vi "Create All Message Queues.vi"(8 "error in (no error)":errorcluster) -> (0 "error out":errorcluster, 3 "Message Queues out":T1)   [LabVIEW 2015, in "Message Queue.lvlib"]
doc: "This VI creates and initializes all the message queues for your application. If your application requires more than one message queue, right-click the \"Message Queues\" constant above and select Open Type Def. Add the new Message Queue(s) to the type definition, then initialize them in this VI."
uses:
  Message Queue.lvlib
  All Message Queues.ctl
  Message Cluster.ctl
  Enqueue Message (Single).vi
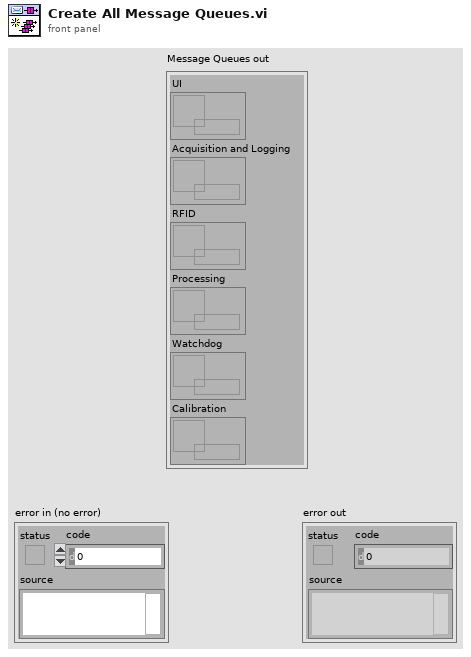
[diagram p1: front panel]
types:
  T1 = typedef "Message Queue.lvlib/All Message Queues.ctl" = cluster{"UI":refnum<queue>, "Acquisition and Logging":refnum<queue>, "RFID":refnum<queue>, "Processing":refnum<queue>, "Watchdog":refnum<queue>, "Calibration":refnum<queue>}
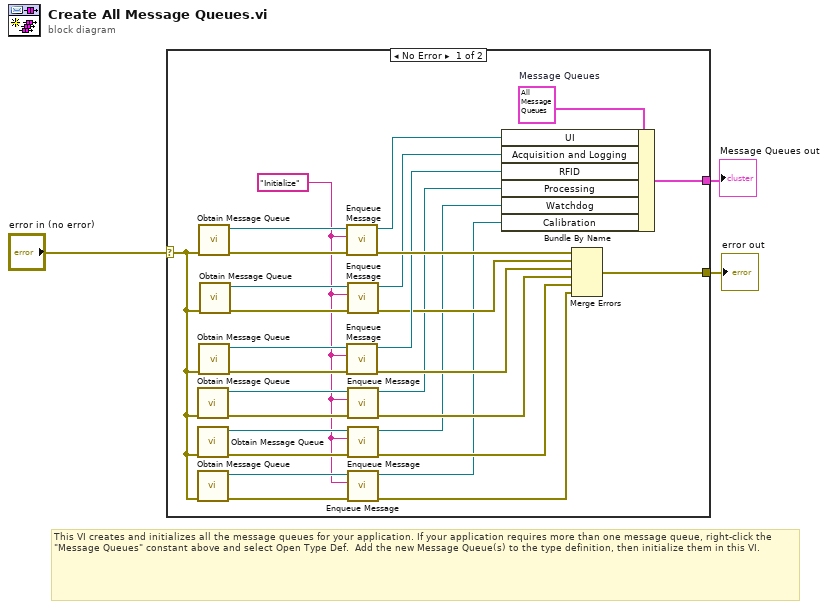
[diagram p0: block diagram]
diagram:
  # "This VI creates and initializes all the message queues for your application. If your application requires more than one message queue, right-click the \"Message Queues\" constant above and select Open Type Def.  Add the new Message Queue(s) to the type definition, then initialize them in this VI."
  n1 = case shown="No Error" "error in (no error)" {
    selector: "error in (no error)" -> [w8 w33]
    tunnel: [w20 w33] -> w3
    tunnel: [w30 _] -> w2
    frame No Error {
      w6 = "Initialize" ("Message")
      w31 = T1 {"UI"=refnum, "Acquisition and Logging"=refnum, "RFID"=refnum, "Processing"=refnum, "Watchdog"=refnum, "Calibration"=refnum}  # Message Queues
      n2 = call "Obtain Message Queue.vi"("error in (no error)"=w8) -> ("error out"=w15:errorcluster, "Message Queue"=w14:refnum<queue>)  [unwired: 9 in]
      n3 = call "Obtain Message Queue.vi"("error in (no error)"=w8) -> ("error out"=w13:errorcluster, "Message Queue"=w10:refnum<queue>)  [unwired: 9 in]
      n4 = call "Obtain Message Queue.vi"("error in (no error)"=w8) -> ("error out"=w9:errorcluster, "Message Queue"=w7:refnum<queue>)  [unwired: 9 in]
      n5 = call "Obtain Message Queue.vi"("error in (no error)"=w8) -> ("error out"=w29:errorcluster, "Message Queue"=w28:refnum<queue>)  [unwired: 9 in]
      n6 = call "Obtain Message Queue.vi"("error in (no error)"=w8) -> ("error out"=w25:errorcluster, "Message Queue"=w24:refnum<queue>)  [unwired: 9 in]
      n7 = call "Obtain Message Queue.vi"("error in (no error)"=w8) -> ("error out"=w26:errorcluster, "Message Queue"=w27:refnum<queue>)  [unwired: 9 in]
      n8 = call-poly "Enqueue Message.vi"("error in (no error)"=w29, "Message"=w6, "Message Queue"=w28) -> ("error out"=w32:errorcluster, "dup Message Queue"=w23:refnum<queue>)  [unwired: 7 in]
      n9 = call-poly "Enqueue Message.vi"("error in (no error)"=w25, "Message"=w6, "Message Queue"=w24) -> ("error out"=w18:errorcluster, "dup Message Queue"=w21:refnum<queue>)  [unwired: 7 in]
      n10 = call-poly "Enqueue Message.vi"("error in (no error)"=w26, "Message"=w6, "Message Queue"=w27) -> ("error out"=w19:errorcluster, "dup Message Queue"=w22:refnum<queue>)  [unwired: 7 in]
      n11 = call-poly "Enqueue Message.vi"("error in (no error)"=w15, "Message"=w6, "Message Queue"=w14) -> ("error out"=w16:errorcluster, "dup Message Queue"=w17:refnum<queue>)  [unwired: 7 in]
      n12 = call-poly "Enqueue Message.vi"("error in (no error)"=w13, "Message"=w6, "Message Queue"=w10) -> ("error out"=w12:errorcluster, "dup Message Queue"=w11:refnum<queue>)  [unwired: 7 in]
      n13 = call-poly "Enqueue Message.vi"("error in (no error)"=w9, "Message"=w6, "Message Queue"=w7) -> ("error out"=w4:errorcluster, "dup Message Queue"=w5:refnum<queue>)  [unwired: 7 in]
      n14 = Bundle By Name(cluster=w31, "UI"=w23, "Acquisition and Logging"=w22, "RFID"=w21, "Processing"=w17, "Watchdog"=w11, "Calibration"=w5) -> (w30:T1)
      n15 = Merge Errors(w32, w19, w18, w16, w12, w4) -> (w20:errorcluster)
    }
    frame Error {
    }
  }
  "Message Queues out" <- w2
  "error out" <- w3
